vi "ex3.vi"() -> ()   [LabVIEW 2022 SP3]
panel:
  in  "Save Button":bool
  in  "stop":bool
  in  "dx [ms]":dbl
  in  "Amplitude":dbl
  out "Sine":dbl(graph)
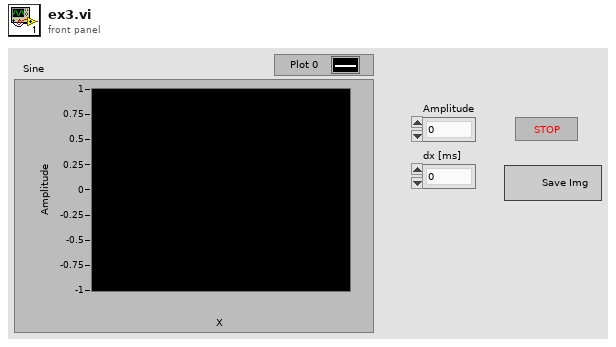
[diagram p1: front panel]
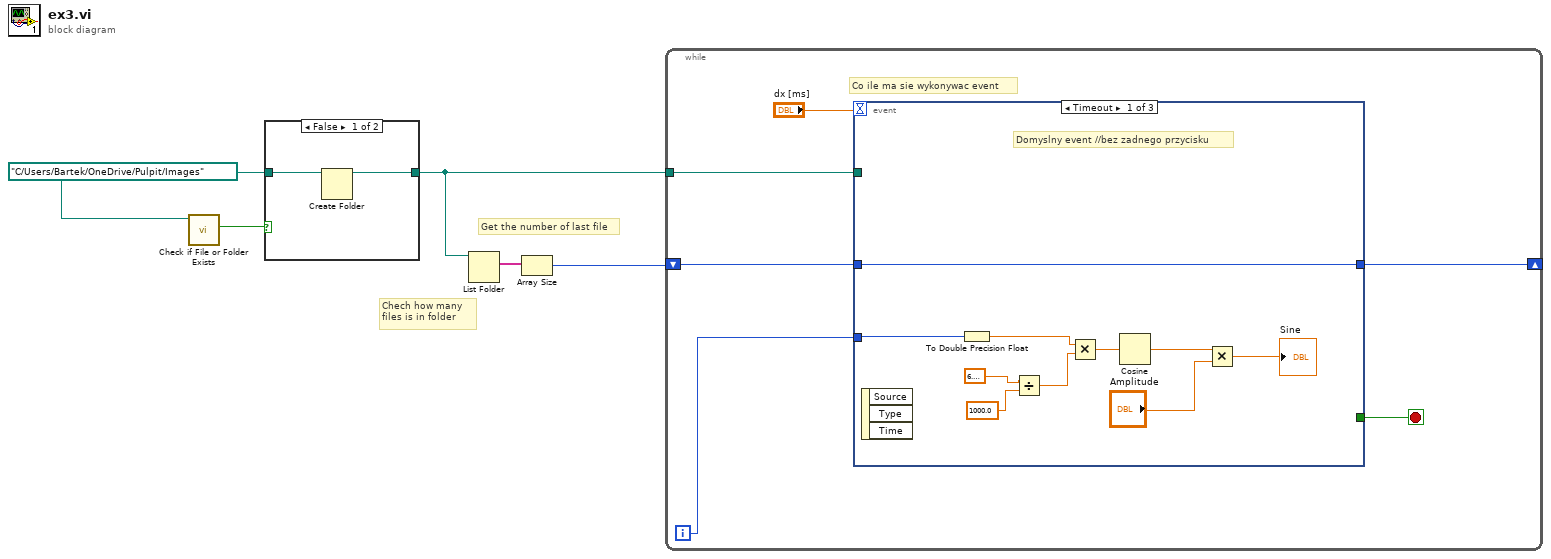
[diagram p0: block diagram]
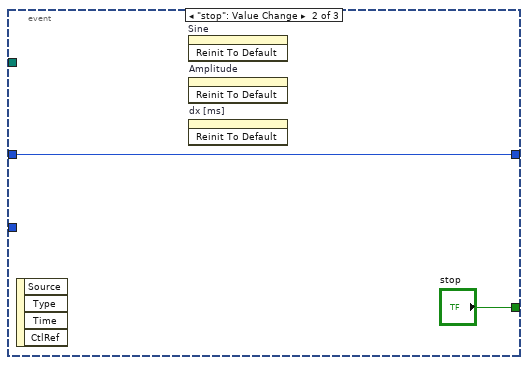
[diagram p2: hidden frame]
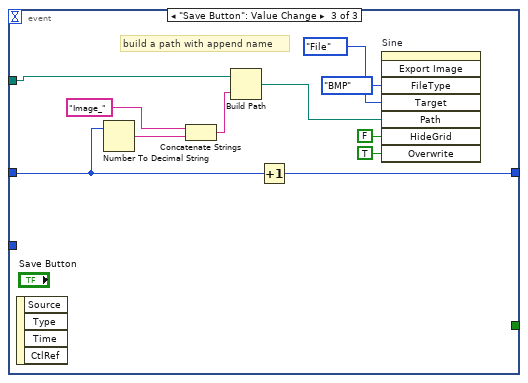
[diagram p3: hidden frame]
diagram:
  w1 = path "C:/Users/Bartek/OneDrive/Pulpit/Images"
  # "Get the number of last file"
  # "Chech how many\nfiles is in folder"
  n1 = call <vilib>:"Check if File or Folder Exists.vi"("path"=w1) -> ("file or folder exists?"=w5:bool)  [unwired: 8 in, 2 out]
  n2 = case shown="False" w5 {
    tunnel: w1 -> [w7 w8]
    tunnel: [w6 w8] -> w3
    frame False {
      n3 = Create Folder(path (use dialog)=w7) -> (created path=w6:path)  [unwired: 2 in, 2 out]
    }
    frame True {
    }
  }
  n4 = List Folder(path=w3) -> (filenames=w4:string[])  [unwired: 3 in, 3 out]
  n5 = Array Size(array=w4) -> (size(s)=w2:i32)
  n6 = while {
    tunnel: w3 -> [w13]
    shift-right: [w11] -> _
    shift-left: w2 -> [w12]
    i -> [w10]
    stop <- w9 stop-if-true
    # "Co ile ma sie wykonywac event"
    n7 = event shown="[0] Timeout" {
      selector: _ -> [_ _ _]
      dyn-events: _ -> [_ _ _]
      timeout: "dx [ms]" -> [_ _ _]
      tunnel: w13 -> [_ _ w33]
      tunnel: w12 -> [w24 w26 w36]
      tunnel: [w24 w26 w37] -> w11
      tunnel: w10 -> [w23 _ _]
      tunnel: [_ "stop" _] -> w9
      event Timeout {
        # "Domyslny event //bez zadnego przycisku"
        n8 = event-data() -> ()  [unwired: 1 in, 3 out]
        n9 = To Double Precision Float(number=w23) -> (double precision float=w22:dbl)
        n10 = Divide(x=6.283185307179586, y=1000.0) -> (x/y=w15:dbl)
        n11 = Multiply(x=w22, y=w15) -> (x*y=w21:dbl)
        n12 = Cosine(x=w21) -> (cos(x)=w20:dbl)
        n13 = Multiply(x=w20, y="Amplitude") -> (x*y=→"Sine":dbl)
      }
      event "stop": Value Change {
        n14 = event-data() -> ()  [unwired: 1 in, 4 out]
        n15 = invoke on="Sine" class="WFChart (strict)" method="Reinit To Default"() -> ()  [unwired: 3 in, 3 out]
        n16 = invoke on="Amplitude" class="DigNum (strict)" method="Reinit To Default"() -> ()  [unwired: 3 in, 3 out]
        n17 = invoke on="dx [ms]" class="DigNum (strict)" method="Reinit To Default"() -> ()  [unwired: 3 in, 3 out]
      }
      event "Save Button": Value Change {
        # "build a path with append name"
        n18 = event-data() -> ()  [unwired: 1 in, 4 out]
        n19 = Number To Decimal String(number=w36) -> (decimal integer string=w35:string)  [unwired: 1 in]
        n20 = Concatenate Strings("Image_" ("string"), w35) -> (w32:string)
        n21 = Build Path(base path=w33, name or relative path=w32) -> (appended path=w30:path)
        n22 = Increment(x=w36) -> (x+1=w37:i32)
        n23 = invoke on="Sine" class="WFChart (strict)" method="Export Image"("FileType"=enum32{"BMP", "EPS", "EMF", "PICT"}."BMP" ("File Type"), "Target"=enum32{"File", "Clipboard"}."File", "Path"=w30, "HideGrid"=FALSE ("Hide Grid"), "Overwrite"=TRUE ("Always Overwrite")) -> ()  [unwired: 3 in, 8 out]
      }
    }
  }
